vi "AlliGator Initialize Internal Variables.vi"(8 "error in (no error)":errorcluster, 9 "Alligator version":string, 10 "State Indicators":refnum<vi>, 11 "Graph References":refnum<vi>[](array[refnum])) -> (0 "error out":errorcluster, 1 "Message":string)   [LabVIEW 2021, in "AlliGator Action Engine.lvlib"]
doc: "Initializes AlliGator internal variables."
uses:
  AlliGator Action Engine.lvlib
  AlliGator State Indicators List.ctl
  AlliGator Variables List.ctl
  Image/Image Zoom Factor.ctl
  AlliGator Skippable Windows Status.ctl
  AlliGator ROI Manager Actions.ctl
  AlliGator Phasor Harmonic Manager Actions.ctl
  AlliGator Image Profile Plot Data.ctl
  Graphs/XY Graph/XY Plot Data.ctl
  AlliGator Displayed Image.ctl
  AlliGator Local Decay Fit Results.ctl
  AlliGator GUI.lvlib
  AlliGator Globals, Variables & Constants.lvlib
  Image/Image.lvlib
  Graphs/XY Graph/XY Graph Add-Ons.lvlib
  AlliGator ROIs.lvlib
  AlliGator Phasor Plot.lvlib
  AlliGator Image Profile Window.lvlib
  AlliGator Source Image.lvlib
  AlliGator Local Decay Window.lvlib
  Strings/Strings.lvlib
  AlliGator Phasor Graph.lvlib
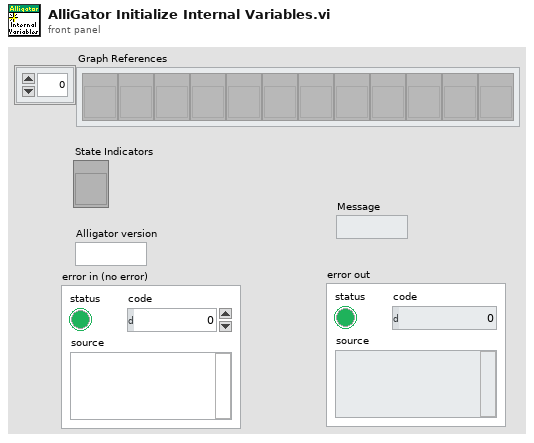
[diagram p1: front panel]
types:
  T1 = typedef "AlliGator Globals, Variables & Constants.lvlib/AlliGator Variables List.ctl" = enum16{"---- GUI ----", "Initialization Status", "State Indicators Refnum", "Original AlliGator Menu Items", "Current Action Loop State", "Script in progress", "Playback", "Loop Playback", "Search ROI Used", "Search ROI", "Decay Graph Max Legend Size", "Intensity Graph Max Legend Size", "Decay Statistics Graph Max Legend Size", "Phasor Graph Max Legend Size", "Phasor Ratio Graph Max Legend Size", "Lifetime Graph Max Legend Size", "---- Files ----", "Export Dataset Frames as Individual Files", "Show Batch Export Help Balloons", "Frames in Dataset", "ptu File Frame Start Indices", "Current Frame in Dataset", "Current Frame Timestamp", "------ Python Plugins ------", "Python Plugins Information", "Python Session", "Valid Python Session?", "---- Source Image ----", "Dataset Loaded", "Dataset Metadata", "Dataset Channel", "Dataset Data Description", "Background Dataset Metadata", "Background Dataset Channel", "Background Dataset Data Description", "Background File Subtraction", "Background File Path", "Background File Pile-up Correction", "Background File Pixel Well Capacity", "Background File Scaling Factor", "Source Image ROIs", "Current Source Image ROI", "Source Image ROI Event Refnum", "X_Source Image Display Range", "X_Source Image Palette Information", "Source Image Palette List", "Source Image Scale", "Current Dataset Load Settings", "Source Image:ROI Overlay Color", "---- Image Profile Window ----", "Image Profile:Overlay ROI in Source Image", "Image Profile Window Event Refnum", "Image Profile:IntensityType", "Image Profile:Intensity Average Type", "Image Profile:Intensity-weighted SDV", "Image Profile:Box Profile Type", "Image Profile Window Open", "Image Profile:Plotted Fit Parameter", "X_Type of Displayed Image", "X_Time Gate Slider", "Dataset Path", "Source Image Overlay to Erase", "Is Displayed Image Accumulated", "White Light Image Modified", "Mask Image Modified", "Macrotime Gate Separation", "------ Phasor Graph -------", "Phasor Graph:Show Line", "---- Phasor Plot ---", "Phasor Plot Parameters Changed", "FLI Dataset Modified since last Phasor Plot Calculation", "Phasor Harmonics Data", "Selected Phasor Harmonics", "Phasor Harmonic Manager Event Refnum", "Phasor Plot ROIs", "Current Phasor Plot ROI", "Phasor Plot ROI Event Refnum", "Phasor Plot Image Reference Points", "Phasor Plot Computed", "Phasor Plot Palette Information", "Phasor Plot Palette List", "Phasor Ratio Palette Information", "Phasor Ratio Palette List", "Phasor Image Scale", "Phasor Plot Image Overlay to Erase", "Phasor Plot Image Elements to Update", "Current Phasor Plot Calculation Parameters", "Current Phasor Calibration Options", "Reset Cumulated Phasor Plot", "Phasor Ratio Reference 1", "Phasor Ratio Lifetime Reference 1", "Phasor Ratio Reference 1 Frequency", "Phasor Ratio Reference 2", "Phasor Ratio Lifetime Reference 2", "Phasor Ratio Reference 2 Frequency", "---- Decay Analysis ----", "Number of Selected Decays to Fit", "LS Fit Results", "LAR Fit Results", "BS Fit Results", "Last Decay Max - Min", "Best Fit Parameters", "Best Fit Parameter Names", "Actual Size X", "Actual Size Y", "Binning X", "Binning Y", "Actual # Gates", "Dataset Number", "Gates to...", "Gates Skipped", "Gates to keep", "Gate Step", "Gate Separation", "Reversed Gates", "Pile-up Correction", "Pixel Well Capacity", "Background Subtracted", "Background Subtraction Method", "Background Definition Range", "Background File (deprecated)", "Number of Dataset Accumulated", "Array of Accumulated Dataset Paths", "Do Averaged Datasets", "Destination File Path", "Process Plot Target", "Use 1/D as Phasor Frequency", "---- Decay Fit Parameter Map -----", "Decay Fit Parameter Map Palette Information", "Decay Fit Parameter Map Palette List", "Local Decay Graph Window Event Refnum", "------- Local Decay Window ---------", "Use normalized IRF for convolution", "----- Miscellaneous ----", "Skippable Dialog Windows Status"}
  T2 = typedef "AlliGator Local Decay Window.lvlib/AlliGator Local Decay Fit Results.ctl" = cluster{"Decay, Fit & Residuals":T3[], "Fit Results":string}
  T3 = typedef "AlliGator Image Profile Window.lvlib/AlliGator Image Profile Plot Data.ctl" = cluster{"Plot Name":string, "Plot":T4}
  T4 = typedef "XY Graph Add-Ons.lvlib/XY Plot Data.ctl" = cluster{"X Array":dbl[], "Y Array":dbl[]}
  T5 = typedef "AlliGator Source Image.lvlib/AlliGator Displayed Image.ctl" = enum16{"Single Gate", "Sum of All Gates", "Max of All Gates", "Min of All Gates", "-", "White Ligth Image", "Mask Image"}
  T6 = typedef "AlliGator Phasor Plot.lvlib/AlliGator Phasor Harmonic Manager Actions.ctl" = enum16{"Undefined", "Delete Current Harmonic", "Delete Multiple Harmonics", "Delete All Harmonics", "Swap Harmonics", "Insert Harmonics", "Rename Current Harmonic", "Store New Harmonic", "Store Multiple Harmonics", "Select Next Harmonic", "Select Previous Harmonic", "Update Phasor Harmonic Manager Window"}
  T7 = typedef "AlliGator ROIs.lvlib/AlliGator ROI Manager Actions.ctl" = enum16{"Undefined", "Delete Current ROI", "Delete All Unselected ROIs", "Delete Multiple ROIs", "Delete All ROIs", "Swap ROIs", "Insert ROI", "Update Current ROI Descriptor", "Rename Current ROI", "Store New ROI", "Store Multiple ROIs", "Select Next ROI", "Select Previous ROI", "Find Selected ROI", "Show All ROIs", "Update ROI Manager Window", "Merge All ROIs", "Unmerge ROI", "Set Selected ROI by ID"}
  T8 = typedef "AlliGator GUI.lvlib/AlliGator Skippable Windows Status.ctl" = cluster{"Dialog Window Name":string, "Is skipped":bool}
  T9 = typedef "Image.lvlib/Image Zoom Factor.ctl" = enum16{"Zoom to Fit", "Zoom to Fit (Keep Aspect Ratio)", "Other Zoom Factor"}
  T10 = typedef "AlliGator Action Engine.lvlib/AlliGator State Indicators List.ctl" = enum16{"Phasor Calibration Defined", "Phasor Calibration Series Defined", "Phasor Calibration Map Defined", "Phasor Reference 1 Defined", "Phasor Reference 2 Defined", "Lifetime Reference 1 Defined", "Lifetime Reference 2 Defined", "Phasor Calibration Used", "Phasor Calibration Series Used", "Phasor Calibration Map Used", "Dataset Update Needed", "Phasor Plot Update Needed", "Reference/IRF Defined", "Individual IRFs Defined"}
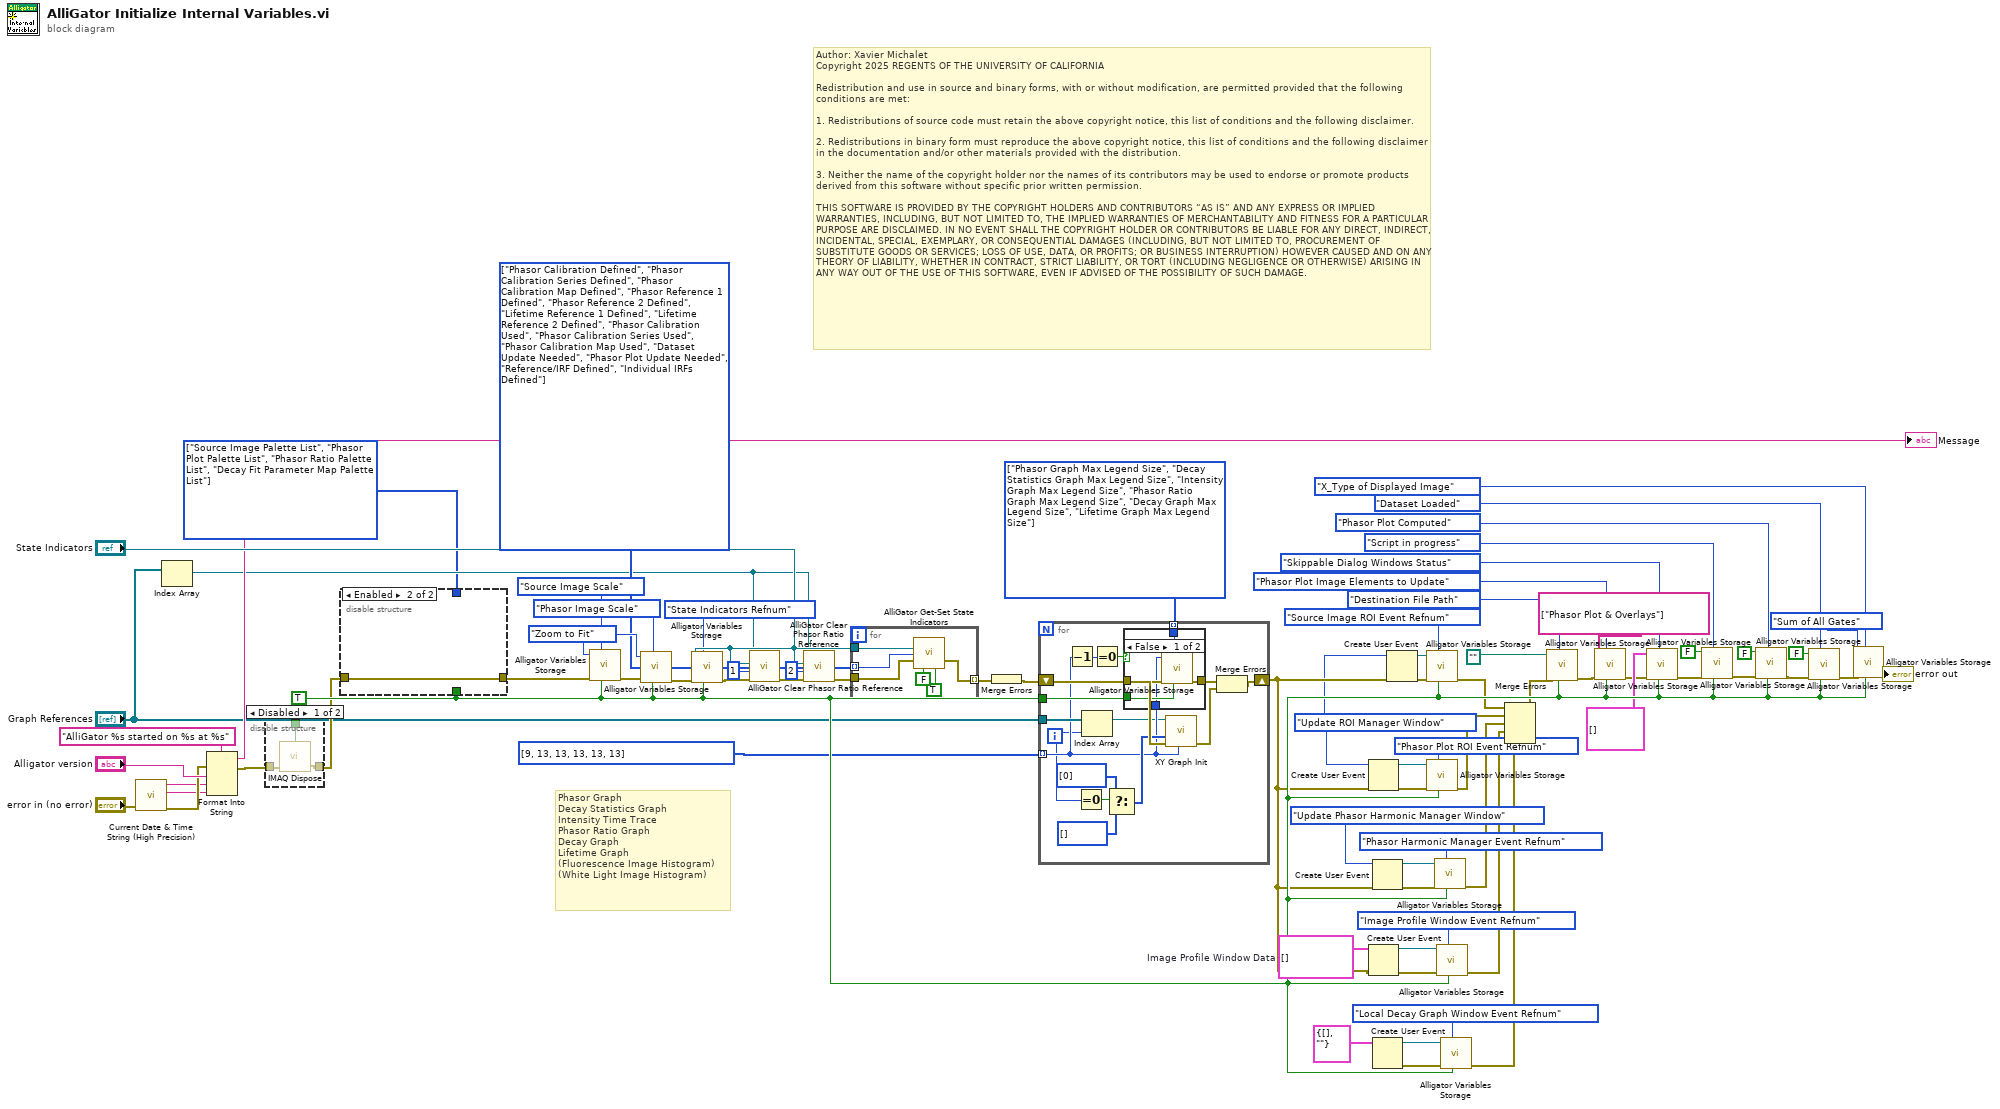
[diagram p0: block diagram]
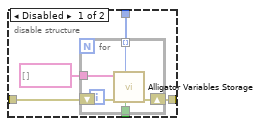
[diagram p2: hidden frame]
diagram:
  w2 = T1[] [enum."Source Image Palette List", enum."Phasor Plot Palette List", enum."Phasor Ratio Palette List", enum."Decay Fit Parameter Map Palette List"] items=["---- GUI ----", "Initialization Status", "State Indicators Refnum", "Original AlliGator Menu Items", "Current Action Loop State", "Script in progress", "Playback", "Loop Playback", "Search ROI Used", "Search ROI", "Decay Graph Max Legend Size", "Intensity Graph Max Legend Size", "Decay Statistics Graph Max Legend Size", "Phasor Graph Max Legend Size", "Phasor Ratio Graph Max Legend Size", "Lifetime Graph Max Legend Size", "---- Files ----", "Export Dataset Frames as Individual Files", "Show Batch Export Help Balloons", "Frames in Dataset", "ptu File Frame Start Indices", "Current Frame in Dataset", "Current Frame Timestamp", "------ Python Plugins ------", "Python Plugins Information", "Python Session", "Valid Python Session?", "---- Source Image ----", "Dataset Loaded", "Dataset Metadata", "Dataset Channel", "Dataset Data Description", "Background Dataset Metadata", "Background Dataset Channel", "Background Dataset Data Description", "Background File Subtraction", "Background File Path", "Background File Pile-up Correction", "Background File Pixel Well Capacity", "Background File Scaling Factor", "Source Image ROIs", "Current Source Image ROI", "Source Image ROI Event Refnum", "X_Source Image Display Range", "X_Source Image Palette Information", "Source Image Palette List", "Source Image Scale", "Current Dataset Load Settings", "Source Image:ROI Overlay Color", "---- Image Profile Window ----", "Image Profile:Overlay ROI in Source Image", "Image Profile Window Event Refnum", "Image Profile:IntensityType", "Image Profile:Intensity Average Type", "Image Profile:Intensity-weighted SDV", "Image Profile:Box Profile Type", "Image Profile Window Open", "Image Profile:Plotted Fit Parameter", "X_Type of Displayed Image", "X_Time Gate Slider", "Dataset Path", "Source Image Overlay to Erase", "Is Displayed Image Accumulated", "White Light Image Modified", "Mask Image Modified", "Macrotime Gate Separation", "------ Phasor Graph -------", "Phasor Graph:Show Line", "---- Phasor Plot ---", "Phasor Plot Parameters Changed", "FLI Dataset Modified since last Phasor Plot Calculation", "Phasor Harmonics Data", "Selected Phasor Harmonics", "Phasor Harmonic Manager Event Refnum", "Phasor Plot ROIs", "Current Phasor Plot ROI", "Phasor Plot ROI Event Refnum", "Phasor Plot Image Reference Points", "Phasor Plot Computed", "Phasor Plot Palette Information", "Phasor Plot Palette List", "Phasor Ratio Palette Information", "Phasor Ratio Palette List", "Phasor Image Scale", "Phasor Plot Image Overlay to Erase", "Phasor Plot Image Elements to Update", "Current Phasor Plot Calculation Parameters", "Current Phasor Calibration Options", "Reset Cumulated Phasor Plot", "Phasor Ratio Reference 1", "Phasor Ratio Lifetime Reference 1", "Phasor Ratio Reference 1 Frequency", "Phasor Ratio Reference 2", "Phasor Ratio Lifetime Reference 2", "Phasor Ratio Reference 2 Frequency", "---- Decay Analysis ----", "Number of Selected Decays to Fit", "LS Fit Results", "LAR Fit Results", "BS Fit Results", "Last Decay Max - Min", "Best Fit Parameters", "Best Fit Parameter Names", "Actual Size X", "Actual Size Y", "Binning X", "Binning Y", "Actual # Gates", "Dataset Number", "Gates to...", "Gates Skipped", "Gates to keep", "Gate Step", "Gate Separation", "Reversed Gates", "Pile-up Correction", "Pixel Well Capacity", "Background Subtracted", "Background Subtraction Method", "Background Definition Range", "Background File (deprecated)", "Number of Dataset Accumulated", "Array of Accumulated Dataset Paths", "Do Averaged Datasets", "Destination File Path", "Process Plot Target", "Use 1/D as Phasor Frequency", "---- Decay Fit Parameter Map -----", "Decay Fit Parameter Map Palette Information", "Decay Fit Parameter Map Palette List", "Local Decay Graph Window Event Refnum", "------- Local Decay Window ---------", "Use normalized IRF for convolution", "----- Miscellaneous ----", "Skippable Dialog Windows Status"] ("Array")
  w61 = T3[] []  # Image Profile Window Data
  w43 = AlliGator_ROI_Manager_Actions."Update ROI Manager Window" ("Action")
  w14 = T1[] [enum."Phasor Graph Max Legend Size", enum."Decay Statistics Graph Max Legend Size", enum."Intensity Graph Max Legend Size", enum."Phasor Ratio Graph Max Legend Size", enum."Decay Graph Max Legend Size", enum."Lifetime Graph Max Legend Size"] items=["---- GUI ----", "Initialization Status", "State Indicators Refnum", "Original AlliGator Menu Items", "Current Action Loop State", "Script in progress", "Playback", "Loop Playback", "Search ROI Used", "Search ROI", "Decay Graph Max Legend Size", "Intensity Graph Max Legend Size", "Decay Statistics Graph Max Legend Size", "Phasor Graph Max Legend Size", "Phasor Ratio Graph Max Legend Size", "Lifetime Graph Max Legend Size", "---- Files ----", "Export Dataset Frames as Individual Files", "Show Batch Export Help Balloons", "Frames in Dataset", "ptu File Frame Start Indices", "Current Frame in Dataset", "Current Frame Timestamp", "------ Python Plugins ------", "Python Plugins Information", "Python Session", "Valid Python Session?", "---- Source Image ----", "Dataset Loaded", "Dataset Metadata", "Dataset Channel", "Dataset Data Description", "Background Dataset Metadata", "Background Dataset Channel", "Background Dataset Data Description", "Background File Subtraction", "Background File Path", "Background File Pile-up Correction", "Background File Pixel Well Capacity", "Background File Scaling Factor", "Source Image ROIs", "Current Source Image ROI", "Source Image ROI Event Refnum", "X_Source Image Display Range", "X_Source Image Palette Information", "Source Image Palette List", "Source Image Scale", "Current Dataset Load Settings", "Source Image:ROI Overlay Color", "---- Image Profile Window ----", "Image Profile:Overlay ROI in Source Image", "Image Profile Window Event Refnum", "Image Profile:IntensityType", "Image Profile:Intensity Average Type", "Image Profile:Intensity-weighted SDV", "Image Profile:Box Profile Type", "Image Profile Window Open", "Image Profile:Plotted Fit Parameter", "X_Type of Displayed Image", "X_Time Gate Slider", "Dataset Path", "Source Image Overlay to Erase", "Is Displayed Image Accumulated", "White Light Image Modified", "Mask Image Modified", "Macrotime Gate Separation", "------ Phasor Graph -------", "Phasor Graph:Show Line", "---- Phasor Plot ---", "Phasor Plot Parameters Changed", "FLI Dataset Modified since last Phasor Plot Calculation", "Phasor Harmonics Data", "Selected Phasor Harmonics", "Phasor Harmonic Manager Event Refnum", "Phasor Plot ROIs", "Current Phasor Plot ROI", "Phasor Plot ROI Event Refnum", "Phasor Plot Image Reference Points", "Phasor Plot Computed", "Phasor Plot Palette Information", "Phasor Plot Palette List", "Phasor Ratio Palette Information", "Phasor Ratio Palette List", "Phasor Image Scale", "Phasor Plot Image Overlay to Erase", "Phasor Plot Image Elements to Update", "Current Phasor Plot Calculation Parameters", "Current Phasor Calibration Options", "Reset Cumulated Phasor Plot", "Phasor Ratio Reference 1", "Phasor Ratio Lifetime Reference 1", "Phasor Ratio Reference 1 Frequency", "Phasor Ratio Reference 2", "Phasor Ratio Lifetime Reference 2", "Phasor Ratio Reference 2 Frequency", "---- Decay Analysis ----", "Number of Selected Decays to Fit", "LS Fit Results", "LAR Fit Results", "BS Fit Results", "Last Decay Max - Min", "Best Fit Parameters", "Best Fit Parameter Names", "Actual Size X", "Actual Size Y", "Binning X", "Binning Y", "Actual # Gates", "Dataset Number", "Gates to...", "Gates Skipped", "Gates to keep", "Gate Step", "Gate Separation", "Reversed Gates", "Pile-up Correction", "Pixel Well Capacity", "Background Subtracted", "Background Subtraction Method", "Background Definition Range", "Background File (deprecated)", "Number of Dataset Accumulated", "Array of Accumulated Dataset Paths", "Do Averaged Datasets", "Destination File Path", "Process Plot Target", "Use 1/D as Phasor Frequency", "---- Decay Fit Parameter Map -----", "Decay Fit Parameter Map Palette Information", "Decay Fit Parameter Map Palette List", "Local Decay Graph Window Event Refnum", "------- Local Decay Window ---------", "Use normalized IRF for convolution", "----- Miscellaneous ----", "Skippable Dialog Windows Status"] ("Array")
  w12 = Image_Zoom_Factor."Zoom to Fit" ("Image Zoom Factor")
  w77 = TRUE ("Get(F)/Set")
  w9 = T10[] [enum."Phasor Calibration Defined", enum."Phasor Calibration Series Defined", enum."Phasor Calibration Map Defined", enum."Phasor Reference 1 Defined", enum."Phasor Reference 2 Defined", enum."Lifetime Reference 1 Defined", enum."Lifetime Reference 2 Defined", enum."Phasor Calibration Used", enum."Phasor Calibration Series Used", enum."Phasor Calibration Map Used", enum."Dataset Update Needed", enum."Phasor Plot Update Needed", enum."Reference/IRF Defined", enum."Individual IRFs Defined"] items=["Phasor Calibration Defined", "Phasor Calibration Series Defined", "Phasor Calibration Map Defined", "Phasor Reference 1 Defined", "Phasor Reference 2 Defined", "Lifetime Reference 1 Defined", "Lifetime Reference 2 Defined", "Phasor Calibration Used", "Phasor Calibration Series Used", "Phasor Calibration Map Used", "Dataset Update Needed", "Phasor Plot Update Needed", "Reference/IRF Defined", "Individual IRFs Defined"] ("Array")
  # "Author: Xavier Michalet\nCopyright 2025 REGENTS OF THE UNIVERSITY OF CALIFORNIA\n\nRedistribution and use in source and binary forms, with or without modification, are permitted provided that the following conditions are met:\n\n1. Redistributions of source code must retain the above copyright notice, this list of conditions and the following disclaimer.\n\n2. Redistributions in binary form must reproduce the above copyright notice, this list of conditions and the following disclaimer in the documentation and/or other materials provided with the distribution.\n\n3. Neither the name of the copyright holder nor the names of its contributors may be used to endorse or promote products derived from this software without specific prior written permission.\n\nTHIS SOFTWARE IS PROVIDED BY THE COPYRIGHT HOLDERS AND CONTRIBUTORS “AS IS” AND ANY EXPRESS OR IMPLIED WARRANTIES, INCLUDING, BUT NOT LIMITED TO, THE IMPLIED WARRANTIES OF MERCHANTABILITY AND FITNESS FOR A PARTICULAR PURPOSE ARE DISCLAIMED. IN NO EVENT SHALL THE COPYRIGHT HOLDER OR CONTRIBUTORS BE LIABLE FOR ANY DIRECT, INDIRECT, INCIDENTAL, SPECIAL, EXEMPLARY, OR CONSEQUENTIAL DAMAGES (INCLUDING, BUT NOT LIMITED TO, PROCUREMENT OF SUBSTITUTE GOODS OR SERVICES; LOSS OF USE, DATA, OR PROFITS; OR BUSINESS INTERRUPTION) HOWEVER CAUSED AND ON ANY THEORY OF LIABILITY, WHETHER IN CONTRACT, STRICT LIABILITY, OR TORT (INCLUDING NEGLIGENCE OR OTHERWISE) ARISING IN ANY WAY OUT OF THE USE OF THIS SOFTWARE, EVEN IF ADVISED OF THE POSSIBILITY OF SUCH DAMAGE."
  # "Phasor Graph\nDecay Statistics Graph\nIntensity Time Trace\nPhasor Ratio Graph\nDecay Graph\nLifetime Graph\n(Fluorescence Image Histogram)\n(White Light Image Histogram)"
  n1 = call "Current Date & Time String (High Precision).vi"("Error In"="error in (no error)") -> ("Error Out"=w69:errorcluster, "time string"=w68:string, "date string"=w67:string)  [unwired: 7 in, 1 out]
  n2 = Index Array(array="Graph References") -> (element=w7:refnum<vi>)  [unwired: 1 in]
  n3 = Format Into String(format string="AlliGator %s started on %s at %s" ("initial string"), error in=w69, "Alligator version", w67, w68) -> (resulting string=→"Message":string, error out=w3:errorcluster)  [unwired: 1 in]
  n4 = disable-structure shown="Disabled" {
    disable-tunnel: [w81 w82] -> w76
    disable-tunnel: w77 -> [w80 _]
    disable-tunnel: w3 -> [w79 w82]
    frame Disabled {
      n5 = call "IMAQ Dispose"("All Images? (No)"=w80, "error in (no error)"=w79) -> ("error out"=w81:errorcluster)  [unwired: 4 in]
    }
    frame Enabled {
    }
  }
  n6 = disable-structure shown="Enabled" {
    disable-tunnel: w77 -> [w87 _]
    disable-tunnel: w76 -> [w86 w93]
    disable-tunnel: w2 -> [w84 _]
    disable-tunnel: [w83 w93] -> w1
    frame Disabled {
      n7 = for {
        tunnel: w87 -> [w92]
        tunnel: string[] [] ("String Array") -> [w90]
        tunnel: w84 -> [w89] mode=indexing
        shift-right: [w88] -> w83
        shift-left: w86 -> [w91]
        n8 = call "Alligator Variables Storage.vi"("Get(F)/Set"=w92, "AlliGator Variable"=w89, "Error In"=w91, "Data in"=w90) -> ("Error Out"=w88:errorcluster)  [unwired: 5 in, 2 out]
      }
    }
    frame Enabled {
    }
  }
  n9 = call "Alligator Variables Storage.vi"("Get(F)/Set"=w77, "AlliGator Variable"=AlliGator_Variables_List."Source Image Scale" ("Alligator Variable"), "Error In"=w1, "Data in"=w12) -> ("Error Out"=w11:errorcluster)  [unwired: 5 in, 2 out]
  n10 = call "Alligator Variables Storage.vi"("Get(F)/Set"=w77, "AlliGator Variable"=AlliGator_Variables_List."Phasor Image Scale" ("Alligator Variable"), "Error In"=w11, "Data in"=w12) -> ("Error Out"=w78:errorcluster)  [unwired: 5 in, 2 out]
  n11 = call "Alligator Variables Storage.vi"("Get(F)/Set"=w77, "AlliGator Variable"=AlliGator_Variables_List."State Indicators Refnum" ("Alligator Variable"), "Error In"=w78, "Data in"="State Indicators") -> ("Error Out"=w71:errorcluster)  [unwired: 5 in, 2 out]
  n12 = call "AlliGator Clear Phasor Ratio Reference.vi"("error in (no error)"=w71, "Reference Number"=1, "State Indicators Refnum"="State Indicators", "Phasor Graph Refnum"=w7) -> ("Error Out"=w72:errorcluster)  [unwired: 7 in]
  n13 = call "AlliGator Clear Phasor Ratio Reference.vi"("error in (no error)"=w72, "Reference Number"=2, "State Indicators Refnum"="State Indicators", "Phasor Graph Refnum"=w7) -> ("Error Out"=w5:errorcluster)  [unwired: 7 in]
  n14 = for {
    tunnel: "State Indicators" -> [w99]
    tunnel: w9 -> [w98] mode=indexing
    tunnel: w5 -> [w96]
    tunnel: [w95] -> w64 mode=indexing
    n15 = call "AlliGator Get-Set State Indicators.vi"("State Indicators Refnum"=w99, "AlliGator State Indicators List"=w98, "Error In"=w96, "ON/OFF"=FALSE ("Set (T)/Unset (F)"), "Set (T)/Get"=TRUE) -> ("Error Out"=w95:errorcluster)  [unwired: 8 in, 2 out]
  }
  n16 = Merge Errors(w64) -> (w6:errorcluster)
  n17 = for {
    tunnel: w14 -> [w115] mode=indexing
    tunnel: w77 -> [w113]
    shift-right: [w110] -> w53
    shift-left: w6 -> [w111]
    tunnel: i32[] [9, 13, 13, 13, 13, 13] ("Max Legend Size (8)") -> [w104] mode=indexing
    tunnel: "Graph References" -> [w112]
    i -> [w100]
    n18 = Decrement(x=w104) -> (x-1=w103:i32)
    n19 = Equal To 0?(x=w100) -> (x = 0?=w108:bool)
    n20 = Index Array(array=w112, index=w100) -> (element=w101:refnum<vi>)
    n21 = Equal To 0?(x=w103) -> (x = 0?=w102:bool)
    n22 = Select(t=i32[] [0] ("Plots to Skip (none)"), s=w108, f=i32[] []) -> (s? t:f=w107:i32[])
    n23 = case shown="False" w102 {
      tunnel: w115 -> [w120 _]
      tunnel: [w119 w121] -> w114
      tunnel: w113 -> [w118 _]
      tunnel: w111 -> [w117 w121]
      tunnel: w104 -> [w116 _]
      frame False {
        n24 = call "Alligator Variables Storage.vi"("Get(F)/Set"=w118, "AlliGator Variable"=w120, "Error In"=w117, "Data in"=w116) -> ("Error Out"=w119:errorcluster)  [unwired: 5 in, 2 out]
      }
      frame True {
      }
    }
    n25 = call "XY Graph Init.vi"("Max Legend Size (8)"=w104, "Error In"=w111, "Plots to Skip (none)"=w107, "XYGraph in"=w101) -> ("Error Out"=w109:errorcluster)  [unwired: 7 in]
    n26 = Merge Errors(w114, w109) -> (w110:errorcluster)
  }
  n27 = Create User Event(user event datatype=w43, error in=w53) -> (user event=w39:refnum<user-event>, error out=w38:errorcluster)
  n28 = Create User Event(user event datatype=w61, error in=w53) -> (user event=w50:refnum<user-event>, error out=w49:errorcluster)
  n29 = Create User Event(user event datatype=AlliGator_Phasor_Harmonic_Manager_Actions."Update Phasor Harmonic Manager Window" ("Action"), error in=w53) -> (user event=w46:refnum<user-event>, error out=w45:errorcluster)
  n30 = Create User Event(user event datatype=T2 {"Decay, Fit & Residuals"=[], "Fit Results"=""} ("Local Decay Fit Results")) -> (user event=w59:refnum<user-event>, error out=w60:errorcluster)  [unwired: 1 in]
  n31 = Create User Event(user event datatype=w43, error in=w53) -> (user event=w16:refnum<user-event>, error out=w17:errorcluster)
  n32 = call "Alligator Variables Storage.vi"("Get(F)/Set"=w77, "AlliGator Variable"=AlliGator_Variables_List."Source Image ROI Event Refnum" ("Alligator Variable"), "Error In"=w17, "Data in"=w16) -> ("Error Out"=w18:errorcluster)  [unwired: 5 in, 2 out]
  n33 = call "Alligator Variables Storage.vi"("Get(F)/Set"=w77, "AlliGator Variable"=AlliGator_Variables_List."Phasor Plot ROI Event Refnum" ("Alligator Variable"), "Error In"=w38, "Data in"=w39) -> ("Error Out"=w41:errorcluster)  [unwired: 5 in, 2 out]
  n34 = call "Alligator Variables Storage.vi"("Get(F)/Set"=w77, "AlliGator Variable"=AlliGator_Variables_List."Phasor Harmonic Manager Event Refnum" ("Alligator Variable"), "Error In"=w45, "Data in"=w46) -> ("Error Out"=w47:errorcluster)  [unwired: 5 in, 2 out]
  n35 = call "Alligator Variables Storage.vi"("Get(F)/Set"=w77, "AlliGator Variable"=AlliGator_Variables_List."Image Profile Window Event Refnum" ("Alligator Variable"), "Error In"=w49, "Data in"=w50) -> ("Error Out"=w52:errorcluster)  [unwired: 5 in, 2 out]
  n36 = call "Alligator Variables Storage.vi"("Get(F)/Set"=w77, "AlliGator Variable"=AlliGator_Variables_List."Local Decay Graph Window Event Refnum" ("Alligator Variable"), "Error In"=w60, "Data in"=w59) -> ("Error Out"=w62:errorcluster)  [unwired: 5 in, 2 out]
  n37 = Merge Errors(w18, w41, w47, w52, w62) -> (w40:errorcluster)
  n38 = call "Alligator Variables Storage.vi"("Get(F)/Set"=w77, "AlliGator Variable"=AlliGator_Variables_List."Destination File Path" ("Alligator Variable"), "Error In"=w40, "Data in"=path "") -> ("Error Out"=w21:errorcluster)  [unwired: 5 in, 2 out]
  n39 = call "Alligator Variables Storage.vi"("Get(F)/Set"=w77, "AlliGator Variable"=AlliGator_Variables_List."Phasor Plot Image Elements to Update" ("Alligator Variable"), "Error In"=w21, "Data in"=string[] ["Phasor Plot & Overlays"] ("element")) -> ("Error Out"=w25:errorcluster)  [unwired: 5 in, 2 out]
  n40 = call "Alligator Variables Storage.vi"("Get(F)/Set"=w77, "AlliGator Variable"=AlliGator_Variables_List."Skippable Dialog Windows Status" ("Alligator Variable"), "Error In"=w25, "Data in"=T8[] []) -> ("Error Out"=w28:errorcluster)  [unwired: 5 in, 2 out]
  n41 = call "Alligator Variables Storage.vi"("Get(F)/Set"=w77, "AlliGator Variable"=AlliGator_Variables_List."Script in progress" ("Alligator Variable"), "Error In"=w28, "Data in"=FALSE ("Get(F)/Set")) -> ("Error Out"=w32:errorcluster)  [unwired: 5 in, 2 out]
  n42 = call "Alligator Variables Storage.vi"("Get(F)/Set"=w77, "AlliGator Variable"=AlliGator_Variables_List."Phasor Plot Computed" ("Alligator Variable"), "Error In"=w32, "Data in"=FALSE ("Set (T)/Unset (F)")) -> ("Error Out"=w35:errorcluster)  [unwired: 5 in, 2 out]
  n43 = call "Alligator Variables Storage.vi"("Get(F)/Set"=w77, "AlliGator Variable"=AlliGator_Variables_List."Dataset Loaded" ("Alligator Variable"), "Error In"=w35, "Data in"=FALSE ("Set (T)/Unset (F)")) -> ("Error Out"=w54:errorcluster)  [unwired: 5 in, 2 out]
  n44 = call "Alligator Variables Storage.vi"("Get(F)/Set"=w77, "AlliGator Variable"=AlliGator_Variables_List."X_Type of Displayed Image" ("Alligator Variable"), "Error In"=w54, "Data in"=AlliGator_Displayed_Image."Sum of All Gates" ("Displayed Image")) -> ("Error Out"=→"error out":errorcluster)  [unwired: 5 in, 2 out]
